vi "AlignedText.vi"(1 "Character Size":sgl, 2 "Color":u32(colorbox), 3 "Alpha":dbl=1.0, 5 "Name":string, 7 "Font Name":string, 9 "Text":string, 11 "error in (no error)":errorcluster, 12 "Font Options":T2) -> (4 "3D Object out":refnum<class "3D Object.lvclass">, 15 "error out":errorcluster)   [LabVIEW 2015, in "3D Object.lvclass"]
uses:
  3D Object.lvclass
  <vilib>/Utility/miscctls.llb/LVSceneTextAlignment.ctl
  <vilib>/picture/3D Picture Control/NI_3D Picture Control.lvlib
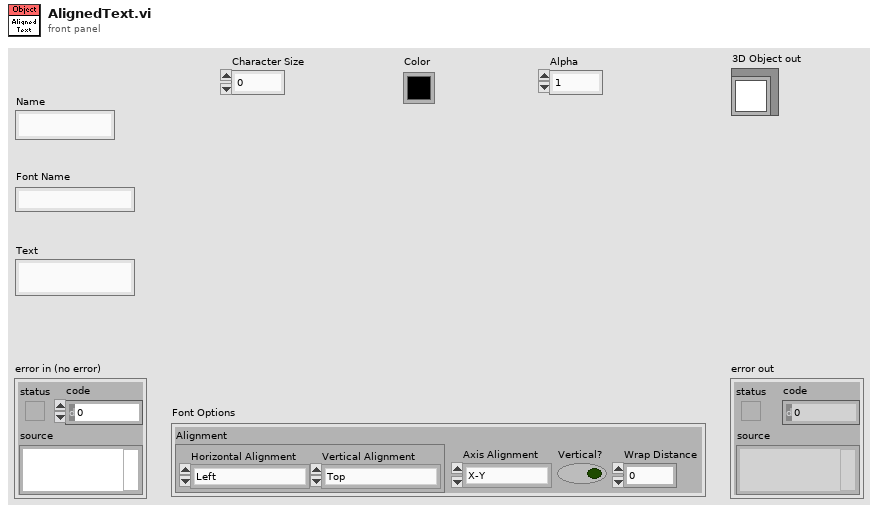
[diagram p1: front panel]
types:
  T1 = typedef "LVSceneTextAlignment.ctl" = cluster{"Horizontal Alignment":enum8{"Left", "Right", "Center"}, "Vertical Alignment":enum8{"Top", "Bottom", "Center", "Base Line", "Bottom Base Line"}}
  T2 = cluster{"Alignment":T1, "Axis Alignment":enum8{"X-Y", "Y-Z", "X-Z", "Reversed X-Y", "Reversed Y-Z", "Reversed X-Z", "Screen"}, "Vertical?":bool, "Wrap Distance":sgl}
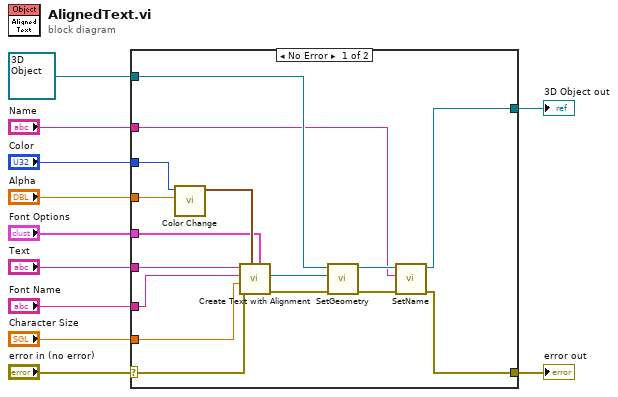
[diagram p0: block diagram]
diagram:
  n1 = case shown="No Error" "error in (no error)" {
    selector: "error in (no error)" -> [w14 w29]
    tunnel: [w13 w29] -> w10
    tunnel: [w12 w28] -> w8
    tunnel: refnum<class "3D Object.lvclass"> refnum ("3D Object in") -> [w27 w28]
    tunnel: "Character Size" -> [w24 _]
    tunnel: "Font Name" -> [w23 _]
    tunnel: "Text" -> [w22 _]
    tunnel: "Alpha" -> [w21 _]
    tunnel: "Color" -> [w20 _]
    tunnel: "Name" -> [w19 _]
    tunnel: "Font Options" -> [w15 _]
    frame No Error {
      n2 = call <vilib>:"Color Change.vi"("Alpha"=w21, "Color"=w20) -> ("RGBA"=w16:cluster{"R":sgl, "G":sgl, "B":sgl, "A":sgl})  [unwired: 9 out]
      n3 = call <vilib>:"Create Text with Alignment.vi"("Font Options"=w15, "Color"=w16, "error in (no error)"=w14, "Character Size"=w24, "Font Name"=w23, "Text"=w22) -> ("error out"=w18:errorcluster, "New Text Refnum"=w26:refnum<vi>)  [unwired: 4 in]
      n4 = call "SetGeometry.vi"("error in (no error)"=w18, "Geometry"=w26, "Object in"=w27) -> ("error out"=w17:errorcluster, "Object out"=w25:refnum<class "3D Object.lvclass">)  [unwired: 7 out]
      n5 = call "SetName.vi"("error in (no error)"=w17, "Name"=w19, "3D Object in"=w25) -> ("error out"=w13:errorcluster, "3D Object out"=w12:refnum<class "3D Object.lvclass">)  [unwired: 7 out]
    }
    frame Error {
    }
  }
  "error out" <- w10
  "3D Object out" <- w8
